vi "Write FXP type.vi"(8 "error in (no error)":errorcluster, 10 "Fixed-Point Representation:Bits":T1, 11 "Fxp Channel in":refnum<class "FPGA Channel.lvclass">) -> (0 "error out":errorcluster, 3 "Fxp Channel out":refnum<class "FPGA Channel.lvclass">)   [LabVIEW 2017, in "FPGA Channel.lvclass"]
uses:
  FPGA Channel.lvclass
  <vilib>/fxp/LVFixedPointRepBitsTypeDef.ctl
  FPGA Channel.lvclass/FPGA Channel.ctl
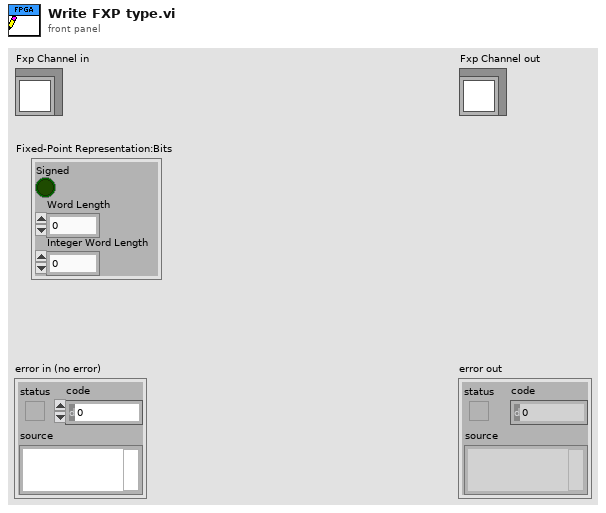
[diagram p1: front panel]
types:
  T1 = typedef "LVFixedPointRepBitsTypeDef.ctl" = cluster{"Signed":bool, "Word Length":u32, "Integer Word Length":i32}
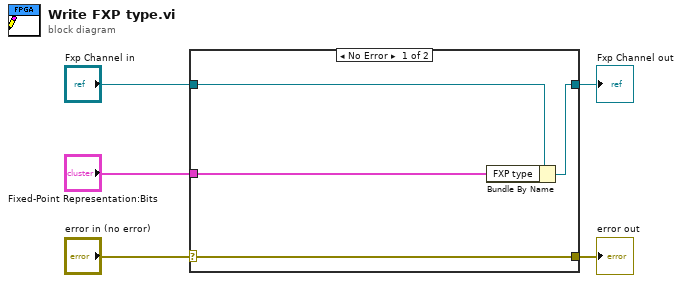
[diagram p0: block diagram]
diagram:
  n1 = case shown="No Error" "error in (no error)" {
    selector: "error in (no error)" -> [w9 w10]
    tunnel: [w9 w10] -> w4
    tunnel: [w7 w11] -> w2
    tunnel: "Fxp Channel in" -> [w8 w11]
    tunnel: "Fixed-Point Representation:Bits" -> [w6 _]
    frame No Error {
      n2 = Bundle By Name(cluster=w8, "FXP type"=w6) -> (w7:refnum<class "FPGA Channel.lvclass">)
    }
    frame Error {
    }
  }
  "error out" <- w4
  "Fxp Channel out" <- w2
